vi "Configure ACLR Measurement.vi"(0 "Spectrum Analyzer in":refnum<class "Spectrum Analyzer.lvclass">, 1 "TX Bandwidth [Hz]":dbl=100.0, 2 "TX Spacing [Hz]":dbl=14000.0, 3 "ALCR Type":enum16{"Relative [dBc]", "Absolute [dBm]"}(ring), 5 "TX Channels":i32=1, 9 "Adj Channels":i32=1, 11 "error in (no error)":errorcluster, 12 "Adj Bandwidth [Hz]":dbl, 13 "Adj Spacing [Hz]":dbl) -> (4 "Spectrum Analyzer out":refnum<class "Spectrum Analyzer.lvclass">, 15 "error out":errorcluster)   [LabVIEW 2020, in "Spectrum Analyzer.lvclass"]
uses:
  Spectrum Analyzer.lvclass
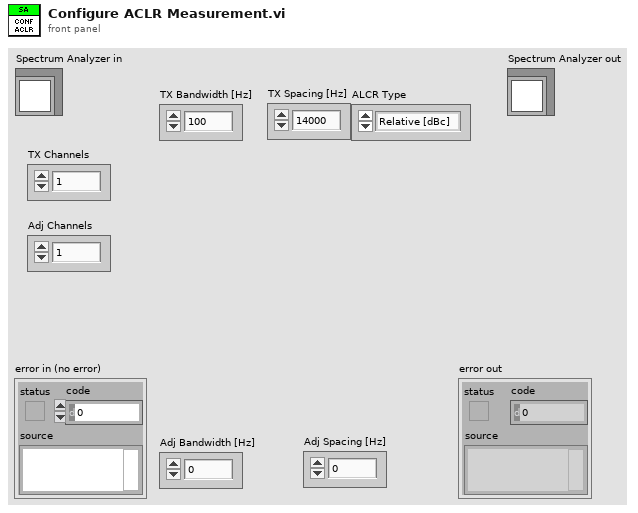
[diagram p1: front panel]
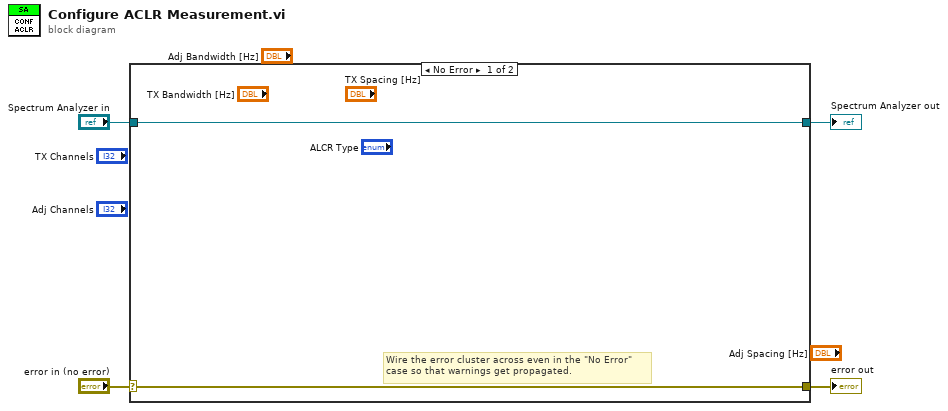
[diagram p0: block diagram]
diagram:
  n1 = case shown="No Error" "error in (no error)" {
    selector: "error in (no error)" -> [w5 w8]
    tunnel: [w5 w8] -> w3
    tunnel: [w6 w7] -> w1
    tunnel: "Spectrum Analyzer in" -> [w6 w7]
    frame No Error {
      # "Wire the error cluster across even in the \"No Error\"\ncase so that warnings get propagated."
    }
    frame Error {
    }
  }
  "error out" <- w3
  "Spectrum Analyzer out" <- w1
